vi "NI VeriStand - Repopulate Nodes in System Explorer.vi"(8 "error in (no error)":errorcluster, 11 "Item Refs in":T1[](array[typedef]) format="%.0x") -> (0 "error out":errorcluster, 3 "Item Refs dup":T1[](array[typedef]) format="%.0x")   [LabVIEW 2020, in "Custom Devices Storage.lvlib"]
doc: "Don't use this VI any more!\nUse instead the version in the Custom Device API.lvlib"
uses:
  Custom Devices Storage.lvlib
  <vilib>/NI VeriStand/Custom Device API/Custom Device Item Ref.ctl
  <vilib>/NI VeriStand/Custom Device API/Custom Device API.lvlib
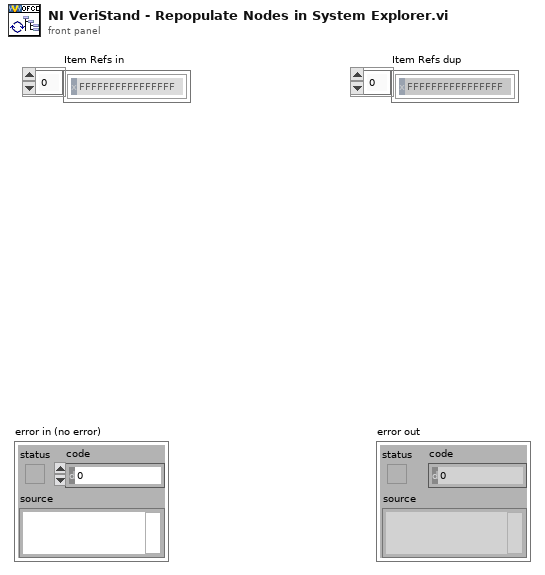
[diagram p1: front panel]
types:
  T1 = typedef "Custom Device API.lvlib/Custom Device Item Ref.ctl" = u64
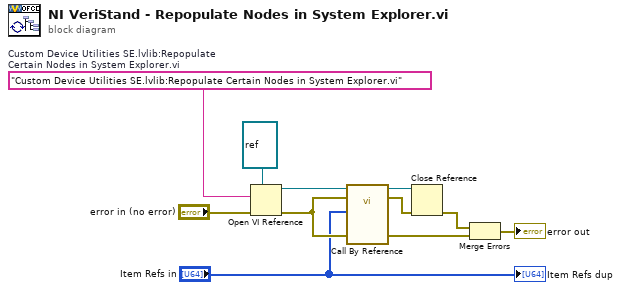
[diagram p0: block diagram]
diagram:
  w11 = "Custom Device Utilities SE.lvlib:Repopulate Certain Nodes in System Explorer.vi"  # Custom Device Utilities SE.lvlib:Repopulate Certain Nodes in System Explorer.vi
  n1 = Open VI Reference(type specifier VI Refnum (for type only)=refnum<vi> refnum, vi path=w11, error in (no error)="error in (no error)") -> (vi reference=w4:refnum<vi>, error out=w5:errorcluster)  [unwired: 3 out]
  n2 = call-by-ref "?"(reference=w4, error in=w5, 8:"error in (no error)"=w5, "Node References"="Item Refs in") -> (reference out=w8:refnum<vi>, error out=w9:errorcluster, 0:"error out"=w10:errorcluster)  [unwired: 9 in]
  n3 = Close Reference(reference=w8, error in (no error)=w9) -> (error out=w7:errorcluster)
  n4 = Merge Errors(w7, w10) -> (→"error out":errorcluster)
  "Item Refs dup" <- "Item Refs in"
